vi "StopSequenceAcqusition.vi"(8 "error in (no error)":errorcluster, 11 "Camera_Prime95B in":refnum<class "Camera_Prime95B.lvclass">) -> (0 "error out":errorcluster, 3 "Camera_Prime95B out":refnum<class "Camera_Prime95B.lvclass">)   [LabVIEW 2020, in "Camera_Prime95B.lvlib" / "Camera_Prime95B.lvclass"]
uses:
  Camera_Prime95B.lvclass
  Camera_Prime95B.lvclass/Camera_Prime95B.ctl
  E:/Development/DevHardSoftware/MMicroscopyAF/Model/Real Hardware/Camera_Prime95B/Camera_Prime95B/Dependencies/PVCamNET.dll
  Dependencies/PVCamNET.dll
  HAL Layer/Component/Camera/Camera/Camera.lvclass
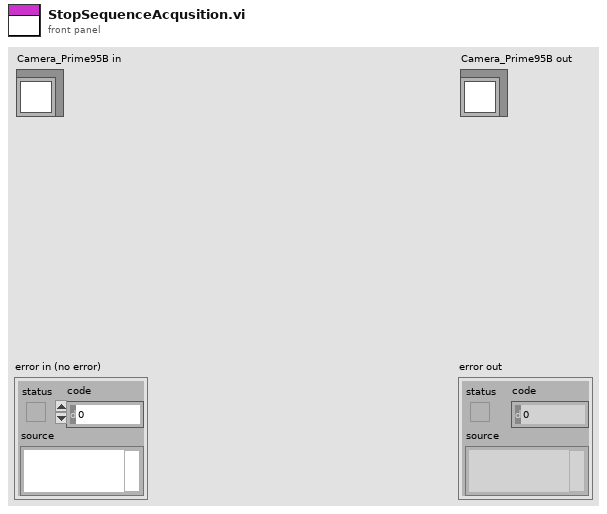
[diagram p1: front panel]
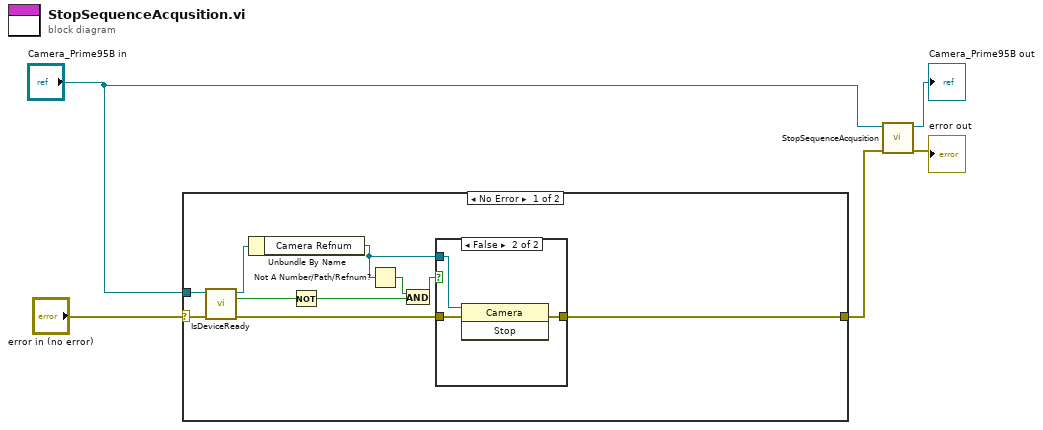
[diagram p0: block diagram]
diagram:
  n1 = case shown="No Error" "error in (no error)" {
    selector: "error in (no error)" -> [w13 w20]
    tunnel: [w15 w20] -> w1
    tunnel: "Camera_Prime95B in" -> [w11 _]
    frame No Error {
      n2 = call-dynamic "IsDeviceReady.vi"("error in (no error)"=w13, "Camera_Prime95B in"=w11) -> ("error out"=w12:errorcluster, "Ready?"=w9:bool, "Camera_Prime95B out"=w10:refnum<class "Camera_Prime95B.lvclass">)  [unwired: 7 in]
      n3 = Unbundle By Name(w10) -> ("Camera Refnum"=w14:refnum<k24>)
      n4 = Not(x=w9) -> (.not. x?=w8:bool)
      n5 = Not A Number/Path/Refnum?(number/path/refnum=w14) -> (NaN/Path/Refnum?=w7:bool)
      n6 = And(x=w7, y=w8) -> (x .and. y?=w6:bool)
      n7 = case shown="False" w6 {
        tunnel: [w16 w19] -> w15
        tunnel: w12 -> [w16 w18]
        tunnel: w14 -> [_ w17]
        frame True {
        }
        frame False {
          n8 = invoke class="Camera" method="Stop"(reference=w17, error in=w18) -> (error out=w19:errorcluster)  [unwired: 1 in, 2 out]
        }
      }
    }
    frame Error {
    }
  }
  n9 = call-parent "StopSequenceAcqusition.vi"("error in (no error)"=w1, "Camera in"="Camera_Prime95B in") -> ("error out"=→"error out":errorcluster, "Camera out"=→"Camera_Prime95B out":refnum<class "Camera_Prime95B.lvclass">)  [unwired: 8 in]
